vi "지진계측기.vi"() -> ()   [LabVIEW 2020]
uses:
  <vilib>/Utility/sysdir.llb/System Directory Type.ctl
panel:
  in  "알람 기준값":dbl format="%#_g M"
  in  "계측 속도":dbl format="%#_g ms"
  out "알람":bool
  in  "프로그램 정지":bool
  in  "알람 리셋":bool
  in  "리히터 저장":bool
  in  "계측 시작":bool
  out "결과 테이블":string[][](array[string])
  out "System Log":string
  out "진도 그래프":dbl[](graph)
  # "리히터 규모 진도 측정 시스템"
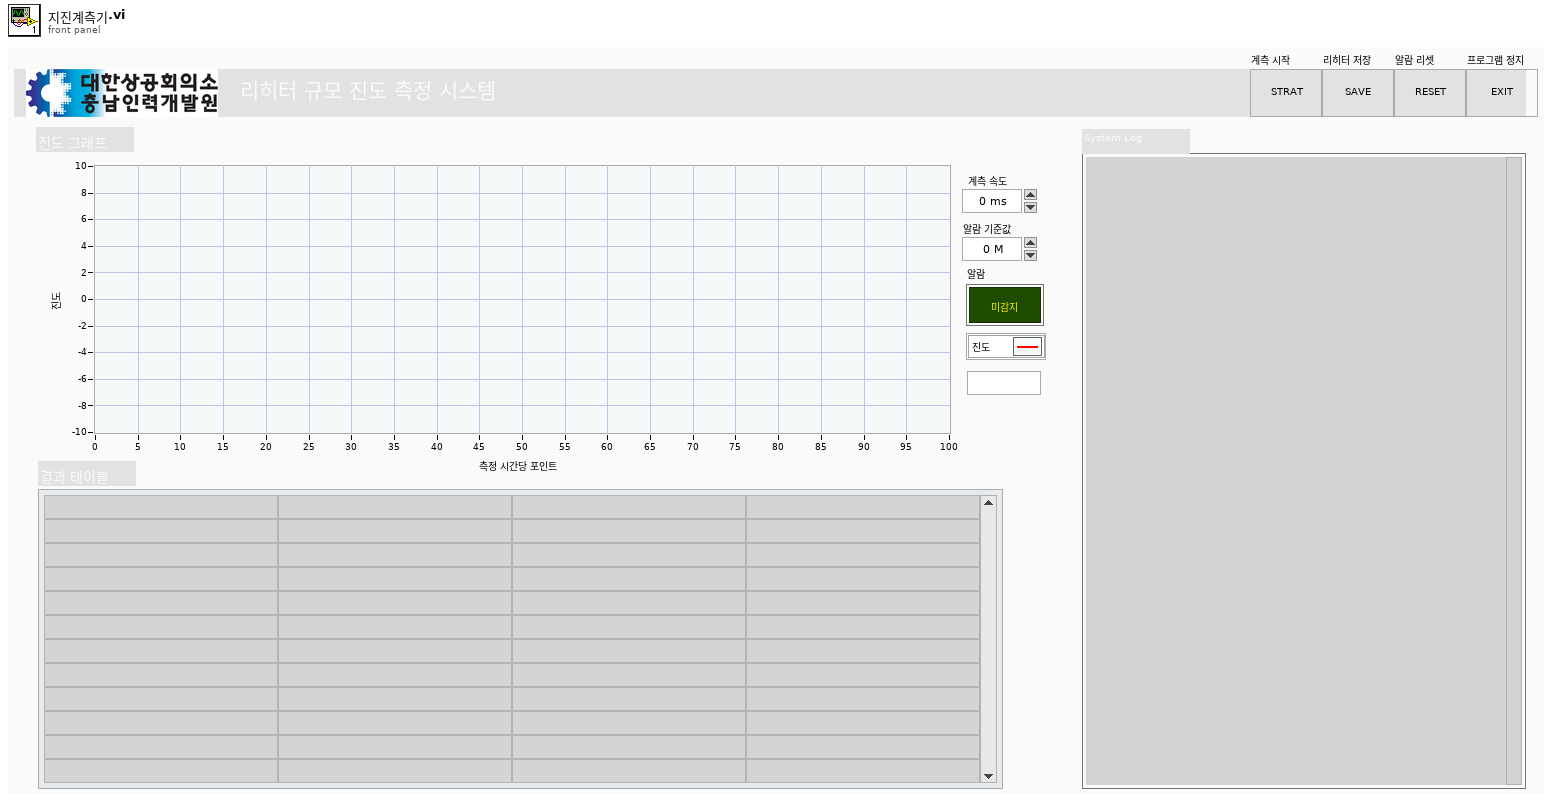
[diagram p1: front panel]
types:
  T1 = cluster{"System Log":string, "진도 그래프":dbl[], "결과 테이블":string[][], "알람":bool, "TDMS이름":string, "도달?":bool}
  T2 = typedef "System Directory Type.ctl" = i32
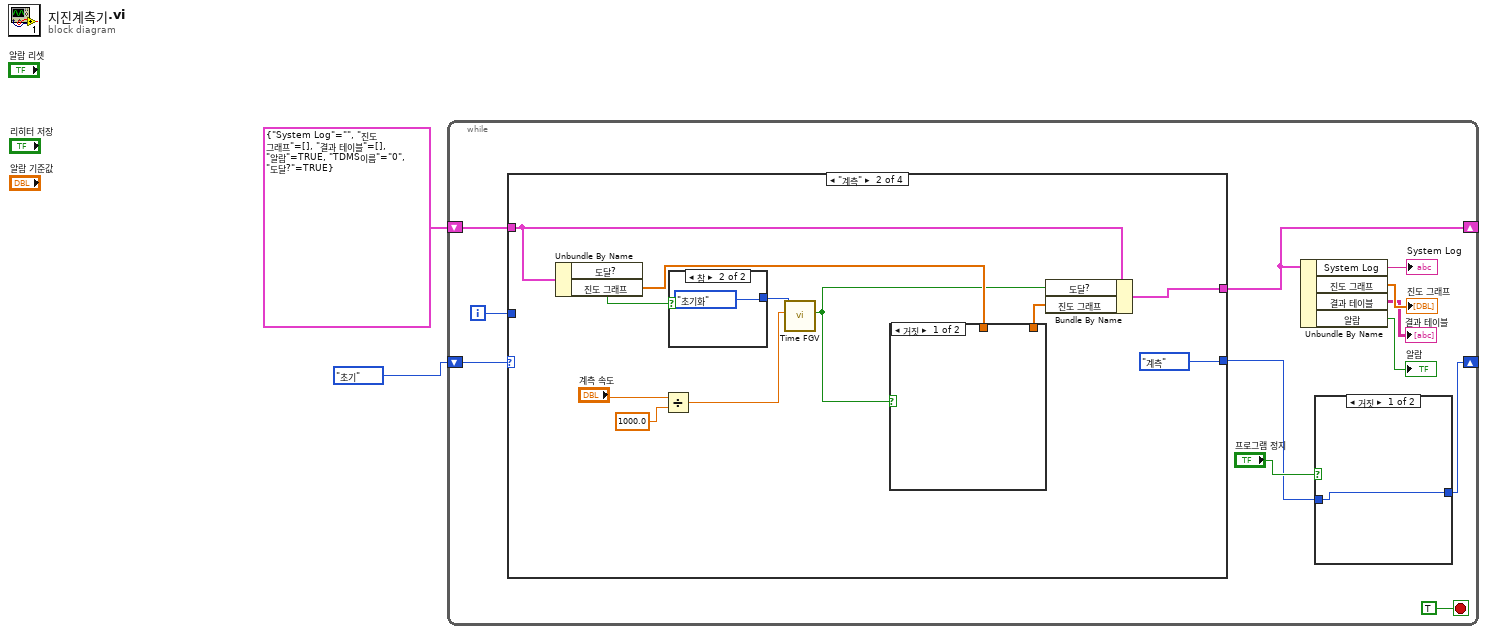
[diagram p0: block diagram]
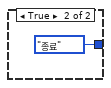
[diagram p2: hidden frame]
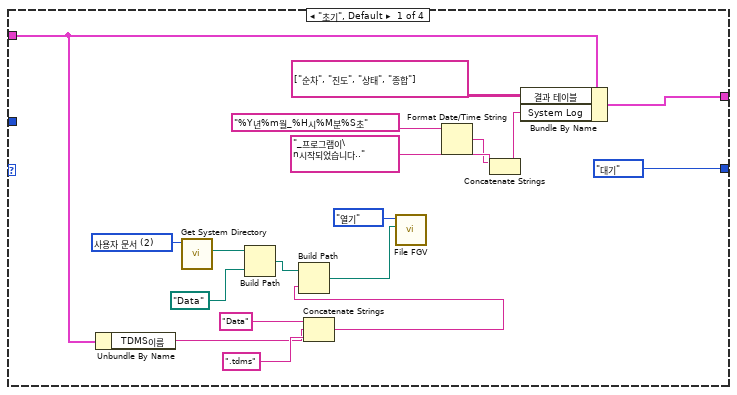
[diagram p3: hidden frame]
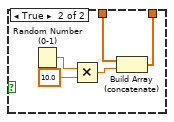
[diagram p4: hidden frame]
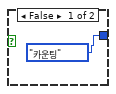
[diagram p5: hidden frame]
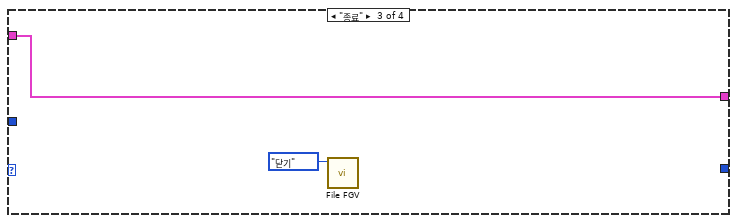
[diagram p6: hidden frame]
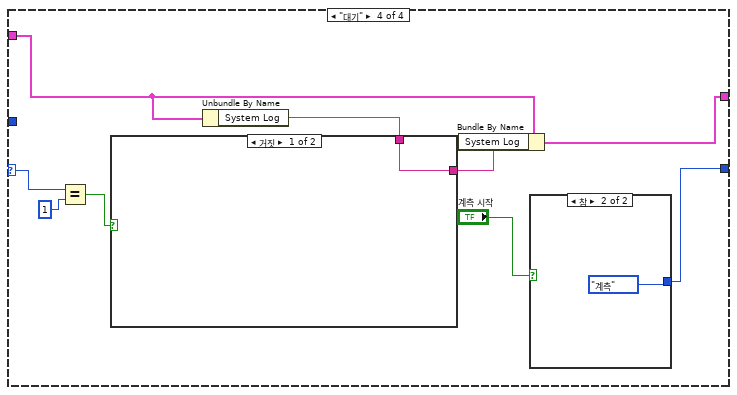
[diagram p7: hidden frame]
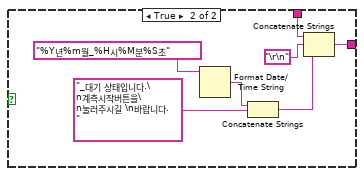
[diagram p8: hidden frame]
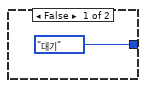
[diagram p9: hidden frame]
diagram:
  n1 = while {
    shift-right: [w4] -> _
    shift-left: enum16{"초기", "대기", "계측", "종료"}."초기" ("열거형") -> [w14]
    shift-right: [w12] -> _
    shift-left: T1 {"System Log"="", "진도 그래프"=[], "결과 테이블"=[], "알람"=TRUE, "TDMS이름"="0", "도달?"=TRUE} -> [w13]
    i -> [w3]
    stop <- TRUE stop-if-true
    n2 = case shown="\"계측\"" w14 {
      selector: w14 -> [_ _ _ w61]
      tunnel: [enum16{"초기", "대기", "계측", "종료"}."대기" ("열거형") enum16{"초기", "대기", "계측", "종료"}."계측" ("열거형") _ w62] -> w5
      tunnel: w13 -> [w24 w42 w54 w57]
      tunnel: [w32 w41 w54 w56] -> w12
      tunnel: w3 -> [_ _ _ _]
      frame "초기", Default {
        w31 = T2 2 items=["사용자 홈"=0, "사용자 데스크탑"=1, "사용자 문서"=2, "사용자 어플리케이션 데이터"=3, "사용자 환경"=4, "사용자 임시"=5, "퍼블릭 문서"=6, "퍼블릭 어플리케이션 데이터"=7, "퍼블릭 환경"=8, "퍼블릭 캐시"=13, "시스템 코어 라이브러리"=9, "시스템 설치된 라이브러리"=10, "어플리케이션 파일"=11, "부팅 볼륨 루트"=12] ("system directory type")
        n3 = Unbundle By Name(w24) -> ("TDMS이름"=w23:string)
        n4 = call <vilib>:"Get System Directory.vi"("system directory type"=w31) -> ("system directory"=w29:path)  [unwired: 10 in]
        n5 = Build Path(base path=w29, name or relative path=path "Data" ("이름 또는 상대 경로")) -> (appended path=w27:path)
        n6 = Concatenate Strings("Data", w23, ".tdms") -> (w22:string)
        n7 = Build Path(base path=w27, name or relative path=w22) -> (appended path=w21:path)
        n8 = call "File FGV.vi"("파일 경로"=w21, "File FGV 상태"=enum16{"열기", "쓰기", "닫기"}."열기") -> ()  [unwired: 10 in]
        n9 = Format Date/Time String(time format string (%c)="%Y년%m월_%H시%M분%S초" ("시간 포맷 문자열 (%c)")) -> (date/time string=w18:string)  [unwired: 2 in]
        n10 = Concatenate Strings(w18, "_프로그램이\n시작되었습니다.." ("시간 포맷 문자열 (%c)")) -> (w17:string)
        n11 = Bundle By Name(cluster=w24, "결과 테이블"=string[][] [["순차", "진도", "상태", "종합"]], "System Log"=w17) -> (w32:T1)
      }
      frame "계측" {
        n12 = Unbundle By Name(w42) -> ("도달?"=w44:bool, "진도 그래프"=w37:dbl[])
        n13 = Divide(x="계측 속도", y=1000.0 ("x/y")) -> (x/y=w38:dbl)
        n14 = case shown="참" w44 {
          tunnel: [enum16{"초기화", "카운팅"}."카운팅" ("Time FGV 상태") enum16{"초기화", "카운팅"}."초기화" ("Time FGV 상태")] -> w43
          frame False {
          }
          frame True {
          }
        }
        n15 = call "Time FGV.vi"("목표 시간"=w38, "Time FGV 상태"=w43) -> ("도달?"=w35:bool)  [unwired: 8 in, 1 out]
        n16 = case shown="거짓" w35 {
          tunnel: w37 -> [_ w47]
          tunnel: [_ w46] -> w36
          frame False {
          }
          frame True {
            n17 = Random Number (0-1)() -> (number: 0 to 1=w50:dbl)
            n18 = Multiply(x=w50, y=10.0) -> (x*y=w48:dbl)
            n19 = Build Array (concatenate)(w47, w48) -> (w46:dbl[])
          }
        }
        n20 = Bundle By Name(cluster=w42, "도달?"=w35, "진도 그래프"=w36) -> (w41:T1)
      }
      frame "종료" {
        n21 = call "File FGV.vi"("File FGV 상태"=enum16{"열기", "쓰기", "닫기"}."닫기") -> ()  [unwired: 11 in]
      }
      frame "대기" {
        n22 = Equal?(x=w61, y=1) -> (x = y?=w55:bool)
        n23 = Unbundle By Name(w57) -> ("System Log"=w59:string)
        n24 = case shown="거짓" w55 {
          tunnel: w59 -> [w64 w66]
          tunnel: [w64 w65] -> w58
          frame False {
          }
          frame True {
            n25 = Format Date/Time String(time format string (%c)="%Y년%m월_%H시%M분%S초" ("시간 포맷 문자열 (%c)")) -> (date/time string=w69:string)  [unwired: 2 in]
            n26 = Concatenate Strings(w69, "_대기 상태입니다.\n계측시작버튼을\n눌러주시길 \n바랍니다." ("시간 포맷 문자열 (%c)")) -> (w67:string)
            n27 = Concatenate Strings(w66, "\r\n", w67) -> (w65:string)
          }
        }
        n28 = Bundle By Name(cluster=w57, "System Log"=w58) -> (w56:T1)
        n29 = case shown="참" "계측 시작" {
          tunnel: [enum16{"초기", "대기", "계측", "종료"}."대기" ("열거형") enum16{"초기", "대기", "계측", "종료"}."계측" ("열거형")] -> w62
          frame False {
          }
          frame True {
          }
        }
      }
    }
    n30 = Unbundle By Name(w12) -> ("System Log"=→"System Log":string, "진도 그래프"=→"진도 그래프":dbl[], "결과 테이블"=→"결과 테이블":string[][], "알람"=→"알람":bool)
    n31 = case shown="거짓" "프로그램 정지" {
      tunnel: w5 -> [w15 _]
      tunnel: [w15 enum16{"초기", "대기", "계측", "종료"}."종료" ("열거형")] -> w4
      frame False {
      }
      frame True {
      }
    }
  }
